vi "Main.vi"() -> ()   [LabVIEW 2024]
doc: "This sample project is built upon the standard state machine template and shows how you could create an application that acquires, analyzes, and presents data. It includes functionality for presenting configuration dialogs, preserving settings between executions, loading and saving data, as well as exporting graph images and text files.\n\nIt is most appropriate for data that is acquired instantly as it does not allow for screen updates mid acquisition nor does it allow for continuous streaming to disk."
uses:
  controls/Vac Graph Config.ctl
  controls/TestCycleParams.ctl
  controls/SurviveCycleParams.ctl
  controls/ControlInput.ctl
  controls/PID Params.ctl
  controls/State.ctl
  <vilib>/Platform/TimedLoop/XDataNode/timing_clust.ctl
  <vilib>/Platform/TimedLoop/XDataNode/nitl_modes.ctl
  <vilib>/Platform/TimedLoop/XDataNode/wakeup.ctl
  <vilib>/platform/TimedLoop/XDataNode/XDataNode.xnode
  <instrlib>/PL Inficon VGC/PL Inficon VGC.lvclass
  <vilib>/Platform/TimedLoop/XDataNode/XDNodeRunTimeDep.lvlib
  <instrlib>/Stanford PTC10/SRS PTC10.lvlib
  <userlib>/_OpenG.lib/time/time.llb/openg_time.lvlib
panel:
  in  "Save Settings on exit":bool=TRUE
  in  "Load Settings":bool
  in  "Save Settings":bool
  out "stopping":bool=TRUE
  in  "Exit":bool
  in  "Main Tabs":enum32{"Setup", "Operating", "ExportData"}(tab)
  in  "Hardware Setup Tabs":T1(tab)=enum."Temperature Control"
  in  "Chamber SP":T2={"mode"=3, "thresholds"={"lower"=0.0001, "upper"=0.0005}, "on"=TRUE} {"thresholds"."upper" format="%#_5e"; "thresholds"."lower" format="%#_5g"; "mode" items=["off", "on", "channel 1", "channel 2", "channel 3"]}
  in  "Backing SP":T2={"mode"=2, "thresholds"={"lower"=1.0, "upper"=5.0}, "on"=TRUE} {"thresholds"."upper" format="%#_5g"; "thresholds"."lower" format="%#_5g"; "mode" items=["off", "on", "channel 1", "channel 2", "channel 3"]}
  out "device information":T3={"type"="VGC503", "model number"="398-483", "serial number"="7433", "firmware version"="1.07", "hardware version"="1.0"}
  out "Cycle Preview":cluster{dbl[], dbl[]}(graph)
  in  "TestCycleParameters":T4={"TAmb"=20.0, "HeaterTestTemp"=-80.0, "HeaterTestDwell"=30, "HeaterTestDuration"=15, "MinOpTemp"=-50.0, "MinOpDwell(min)"=30, "TestHeatingRate (deg/min)"=0.4, "SurviveCycleParameters"={"MinSurviveTemp"=-131.5, "MinSurvive Dwell"=10, "MaxOpTemp"=50.0, "MaxOpDwell"=30, "ControlInput"=2, "ColdStandOff"=4.0, "HotStandoff"=5.0, "SteadyPWM"=20, "MaxCoolingRate (deg/min)"=3.75, "MaxHeatingRate (deg/min)"=2.5}, "CycleType"=0} {"CycleType" items=["Survival", "Operational"]; "SurviveCycleParameters"."SteadyPWM" min=0 max=100 step=1; "SurviveCycleParameters"."ControlInput" items=["3A", "3B", "3C", "3D", "4A", "4B", "4C", "4D"]}
  in  "PTC setup Tabs":enum32{"Macros", "Channels"}(tab)
  in  "PTC Macro Tabs":T7(tab)=enum."ToAmbient"
  out "pwmloop":string="define pwmloop(#t=0 while (1) {waitforsample if(#pwm=0){relays=0}else{if(#t<#pwm) {relays=1}else{relays=3}}#t+=1 if  (#t>99){#t=0} pause 0.2 s})"
  out "Stat1":bool=TRUE
  out "onecycle Macro":string="define onecycle (pwm=100 run pwmloop 5A.PID.Setpoint=-130.0 5A.PID.input=3C while(#3C>-129.0){pause 0.2 s}pwm=10 pause 100 min pwm=0  5A.PID.SetPoint=50.0 while(#3C<49.0){pause 0.2 s} pause 10 min kill pwmloop)"
  out "Stat2":bool=TRUE
  out "control":string="define control (while (#Cycles>0) {onecycle pause 1 s #Cycles-=1})"
  out "Stat3":bool=TRUE
  out "HeatDrive":string="define Failsafe (while(1) {if (#Check <-20){pwm=0 relays=0 outputEnable Off}else{if(#Check>20){pwm=0 relays=0 outputEnable Off}} pause 1 s})"
  out "Stat4":bool=TRUE
  out "ToAmbient":string="define Failsafe (while(1) {if (#Check <-20){pwm=0 relays=0 outputEnable Off}else{if(#Check>20){pwm=0 relays=0 outputEnable Off}} pause 1 s})"
  out "Stat5":bool=TRUE
  in  "TAmbient":dbl=20.0 min=0.0 max=30.0
  in  "AmbientTolerance":dbl=5.0
  out "Startup Code":string
  in  "PTC Channels":enum32{"Heater Output", "Alarm"}(tab)
  out "Control Input":string
  in  "PID Params":T8={"P"=1.14, "I"=0.012, "D"=21.68} {"D" min=0.0; "I" min=0.0; "P" min=0.0}
  in  "Send to PTC":bool
  out "Response":string
  in  "Command":string
  out "PTC10 Info":T9={"Manufacturer"="Stanford Research Systems", "Instrument"=" PTC10 Programmable Temperature Controller", "Serial Number"=" 153826", "Firmware"=" version 4.56"}
  out "Event log":string
  in  "Enable":bool
  in  "Log Interval (s)":dbl=5.0 min=0.1 max=100.0
  in  "LogFile":path=path "C:/Users/Public/Documents/TVC Logs/platten1.xlsx"
  out "Application:Kind":T10(ring)
  out "App Version":string
  out "CycleNumber":i32
  in  "ToTarget":bool
  in  "Target":dbl
  in  "Start":bool
  in  "Cycles to \nPerform":i32=1 min=1 max=1000 step=1
  out "Current \nTarget\nTemperature":dbl=50.0
  in  "Operating Tabs":enum32{"Vacuum", "Temperatures", "Heater Drive"}(tab)
  out "Pressures":waveform(dbl)[](graph)
  out "Backing Good":bool=TRUE
  out "Chamber Good":bool=TRUE
  in  "Vacuum Graph config":T11={"Log/Lin"=TRUE, "Show Backing"=TRUE, "Show Chamber"=TRUE}
  in  "Clear Vacuum Chart":bool
  in  "Clear Charts":bool
  out "Temperature Chart":dynamicdata(graph)
  out "Heater Drive":waveform(dbl)(graph)
  out "Cycles Remaining":i16=1 caption="Cycles\nRemaining"
  out "Relays":T12
  out "Relay wfm":waveform(dbl)
  out "TVC_temperatures_wfm":waveform(dbl)[](array[waveform])
  out "TVC_Temperatures":dbl[](array[numeric])
  out "Status Bar":string="Application exit."
  # "The FileSafe macro looks at the \"Check\" channel every second.\nIf the value is greater than 20, the macro with disable outputs and switch off the cold head."
  # "The heater output channel (5A) provides an analog control voltage\nto the constant current programming input on the CPX400SA \npower supply.\n\nThe Control Input is the RTD input channel that controls the PID loop.\n\nSetup so that 2V output(maximum) corresponds to approx 4A\nof heater current.\n\nSet PID parameters"
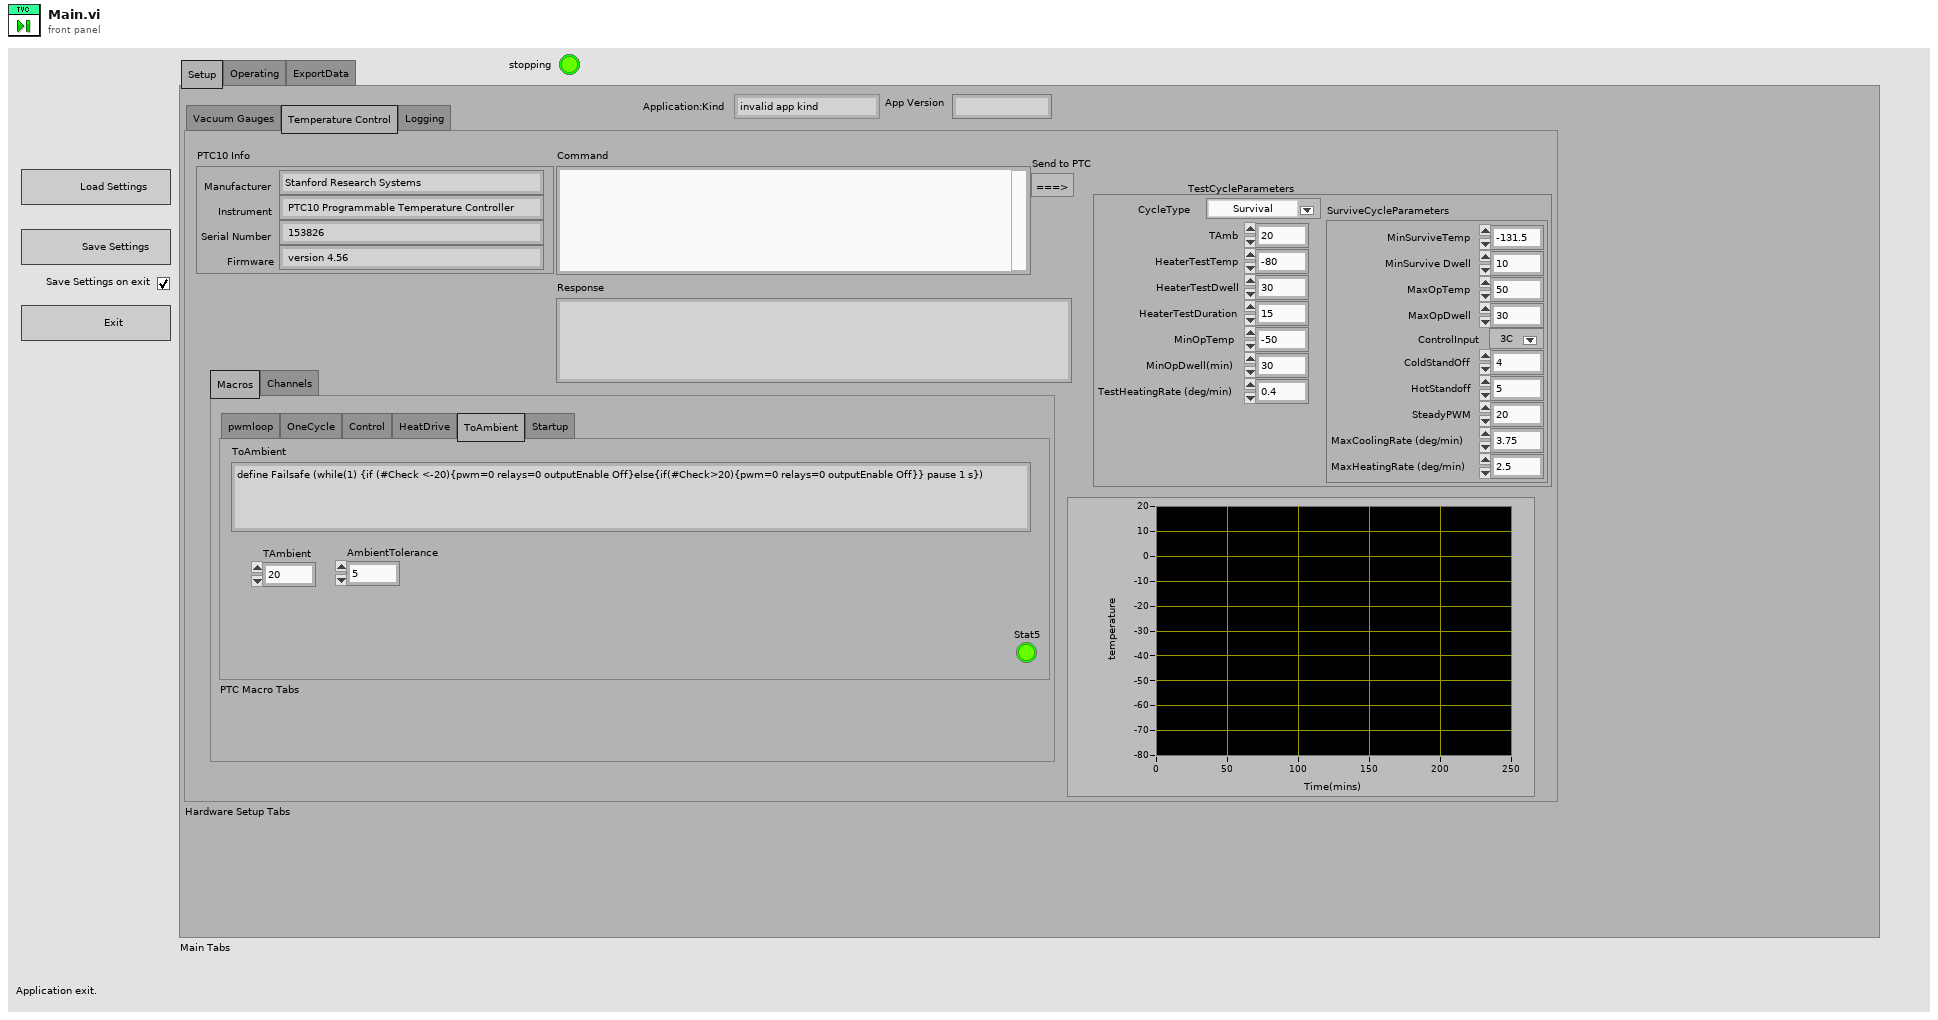
[diagram p1: front panel]
types:
  T1 = enum32{"Vacuum Gauges", "Temperature Control", "Logging"}
  T2 = cluster{"mode":u16, "thresholds":cluster{"lower":dbl, "upper":dbl}, "on":bool}
  T3 = cluster{"type":string, "model number":string, "serial number":string, "firmware version":string, "hardware version":string}
  T4 = typedef "TestCycleParams.ctl" = cluster{"TAmb":dbl, "HeaterTestTemp":dbl, "HeaterTestDwell":i32, "HeaterTestDuration":i32, "MinOpTemp":dbl, "MinOpDwell(min)":i32, "TestHeatingRate (deg/min)":dbl, "SurviveCycleParameters":T5, "CycleType":u16}
  T5 = typedef "SurviveCycleParams.ctl" = cluster{"MinSurviveTemp":dbl, "MinSurvive Dwell":i32, "MaxOpTemp":dbl, "MaxOpDwell":i32, "ControlInput":T6, "ColdStandOff":dbl, "HotStandoff":dbl, "SteadyPWM":i32, "MaxCoolingRate (deg/min)":dbl, "MaxHeatingRate (deg/min)":dbl}
  T6 = typedef "ControlInput.ctl" = u16
  T7 = enum32{"pwmloop", "OneCycle", "Control", "HeatDrive", "ToAmbient", "Startup"}
  T8 = typedef "PID Params.ctl" = cluster{"P":dbl, "I":dbl, "D":dbl}
  T9 = cluster{"Manufacturer":string, "Instrument":string, "Serial Number":string, "Firmware":string}
  T10 = enum32{"invalid app kind", "Development System", "Run Time System", "Student Edition", "Embedded LabVIEW", "Evaluation", "Custom"}
  T11 = typedef "Vac Graph Config.ctl" = cluster{"Log/Lin":bool, "Show Backing":bool, "Show Chamber":bool}
  T12 = cluster{"Sys ON":bool, "Cold Pause":bool, "Alarm":bool}
  T13 = typedef "State.ctl" = enum16{"Initialize", "InitHardware", "WritePTCCode", "CodeToPTC", "Wait for Event", "Update UI", "Save Settings", "Load Settings", "ShutDownHardware", "Exit"}
  T14 = typedef "Data.ctl" = cluster{"UI References":T15, "User Specified":T16}
  T15 = typedef "UI References.ctl" = cluster{"Exit Ref":refnum<vi>, "Save Ref":refnum<vi>, "Export Ref":refnum<vi>, "Acquire Ref":refnum<vi>, "Configure Ref":refnum<vi>, "Graph Ref":refnum<vi>, "Analyze Ref":refnum<vi>, "Status Ref":refnum<vi>, "Snapshot Ref":refnum<vi>, "Start Ref":refnum<vi>}
  T16 = typedef "User Specified Data.ctl" = cluster{"Hardware Configuration":T17, "Vacuum Graph config":T11}
  T17 = typedef "HW Configuration.ctl" = cluster{"VGC50":T18, "PTC10":T19}
  T18 = typedef "VGC50.ctl" = cluster{"serial settings":cluster{"port":refnum<visa-resource-name>, "baud rate":u32}, "device information":cluster{"type":string, "model number":string, "serial number":string, "firmware version":string, "hardware version":string}, "VGC":refnum<class "PL Inficon VGC.lvclass">, "Backing SP":cluster{"mode":u16, "thresholds":cluster{"lower":dbl, "upper":dbl}, "on":bool}, "Chamber SP":cluster{"mode":u16, "thresholds":cluster{"lower":dbl, "upper":dbl}, "on":bool}}
  T19 = typedef "SRS PTC10.ctl" = cluster{"serial settings":cluster{"port":refnum<visa-resource-name>, "baud rate":u32}, "PTC10 Info":cluster{"Manufacturer":string, "Instrument":string, "Serial Number":string, "Firmware":string}, "VISA resource name":refnum<visa-resource-name>, "pwmloop":string, "onecycle":string, "control":string, "HeatDrive":string, "ToAmbient":string, "StartupCode":string, "LogChannels":string[], "Heater O/P Channel":string, " Control Input":string, "TAmbient":dbl, "AmbientTolerance":dbl, "TestCycleParameters":T4, "PID Params":T8}
  T20 = enum8{"Expect success", "Expect error", "Don't check for err"}
  T21 = cluster{"Boolean array[0]":bool, "Boolean array[1]":bool, "Boolean array[2]":bool}
  T22 = typedef "XDNodeRunTimeDep.lvlib/timing_clust.ctl" = cluster{"Expected End [f-1]":u64, "Actual End [f-1]":u64, "Finished Late? [f-1]":bool, "Expected End [i-1]":u64, "Actual End [i-1]":u64, "Finished Late? [i-1]":bool, "Expected Start [i]":u64, "Actual Start [i]":u64, "Expected Start [f]":u64, "Actual Start [f]":u64, "Source Name":string, "Structure Name":string, "Period":i64, "Deadline":i64, "Offset":i64, "Start":i64, "Priority":i32, "Timeout":i32, "Mode":T23, "Wakeup Reason":T24, "Error":errorcluster, "Source Type":string, "Secondary Source Type":string, "Global End Time":u64, "Global Start Time":u64, "Frame Duration":u64, "Iteration Duration":u64, "Assigned CPU":i32, "I/O Scan Engine Mode":u32}
  T23 = typedef "XDNodeRunTimeDep.lvlib/nitl_modes.ctl" = enum32{"No Change", "Process missed periods, maintain original phase", "Discard missed periods, maintain original phase", "Process missed periods, ignore original phase", "Discard missed periods, ignore original phase"}
  T24 = typedef "XDNodeRunTimeDep.lvlib/wakeup.ctl" = enum32{"Normal", "Aborted", "Asynchronous wakeup", "Timing source error", "Timed loop error", "Timeout"}
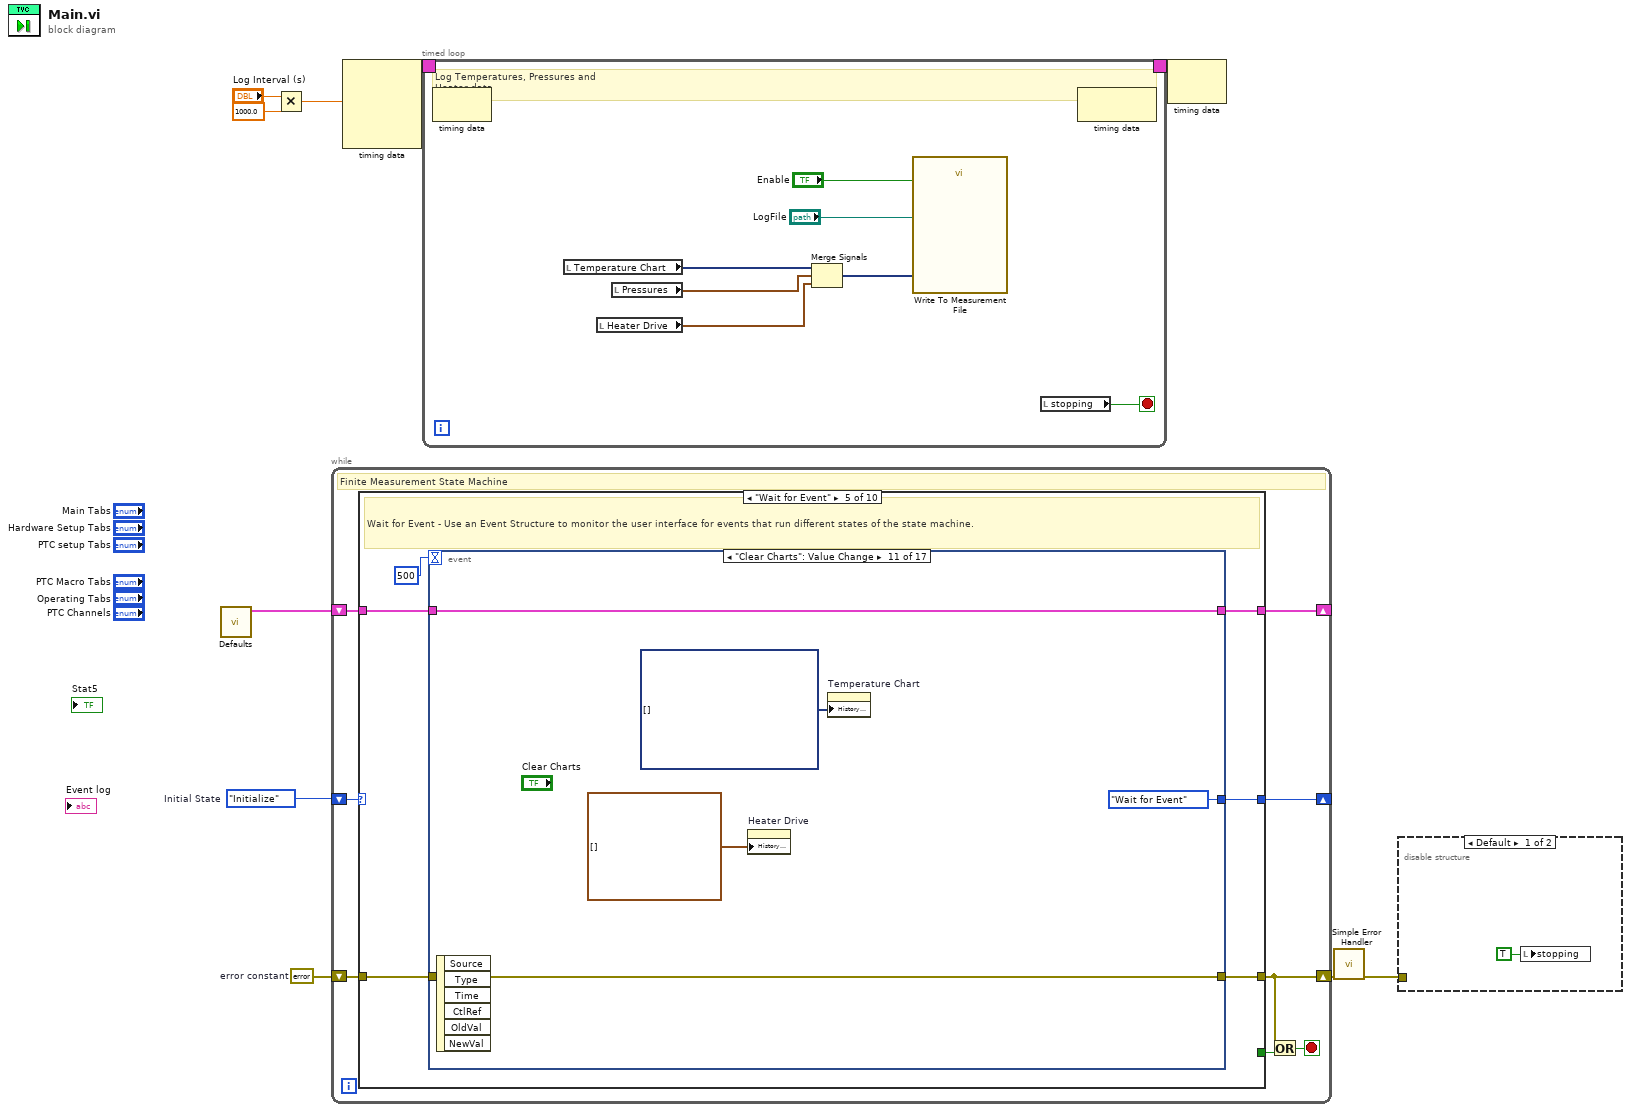
[diagram p0: block diagram]
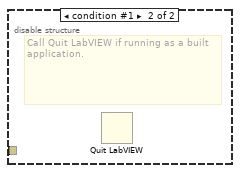
[diagram p2: hidden frame]
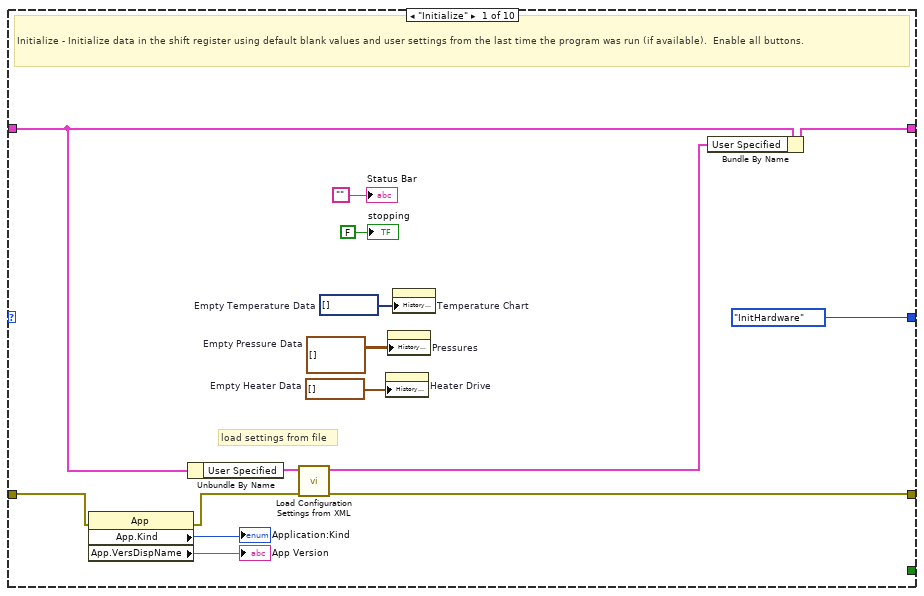
[diagram p3: hidden frame]
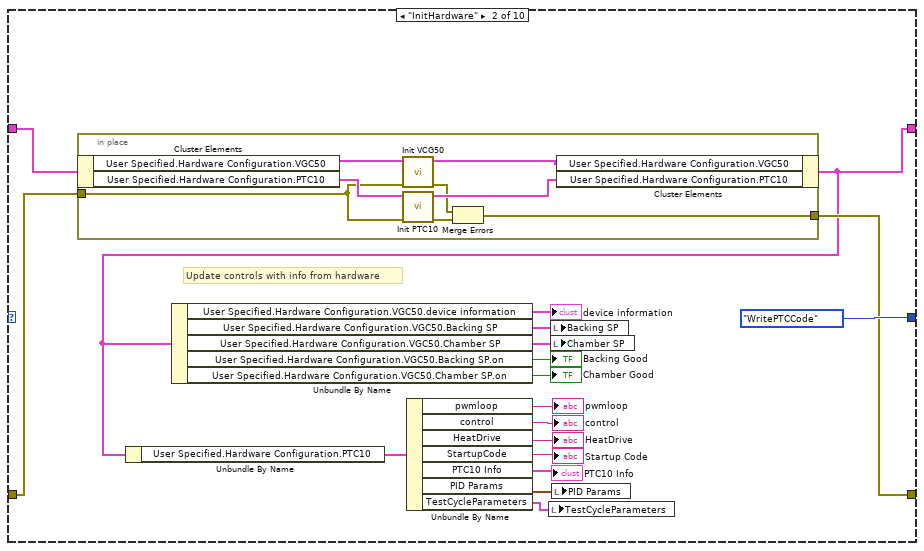
[diagram p4: hidden frame]
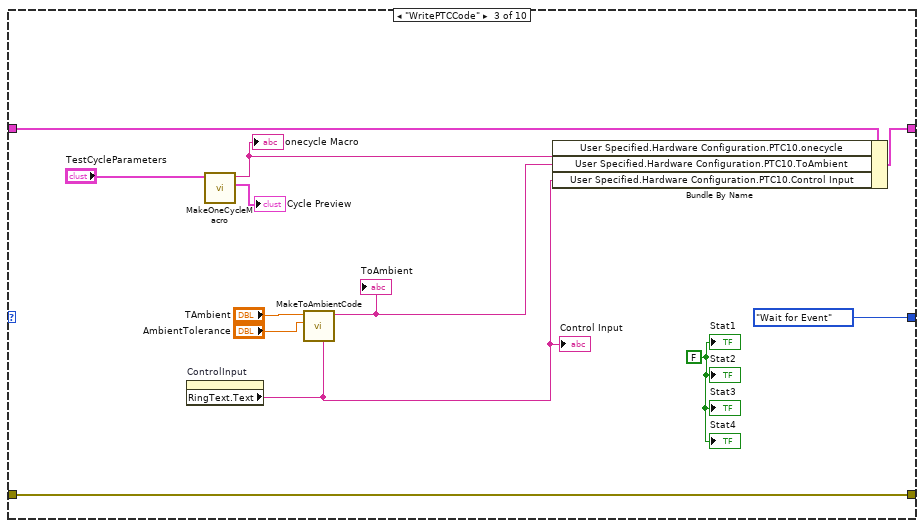
[diagram p5: hidden frame]
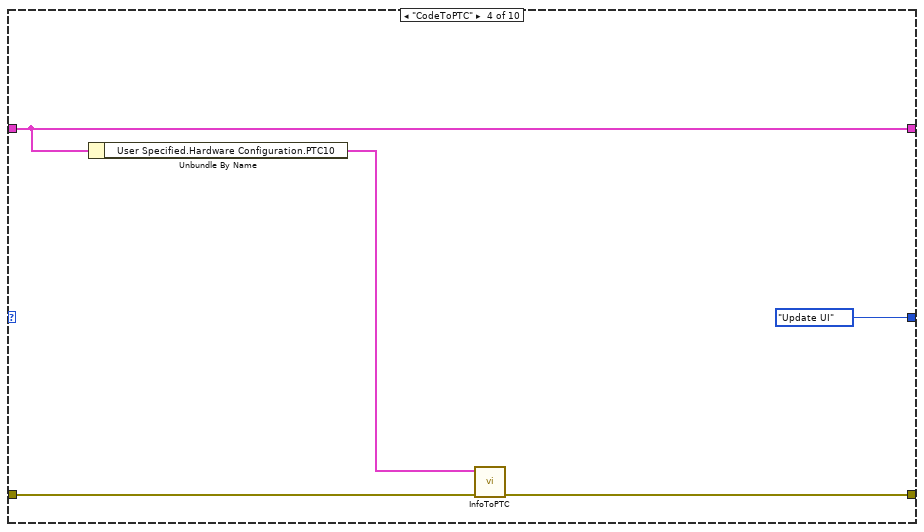
[diagram p6: hidden frame]
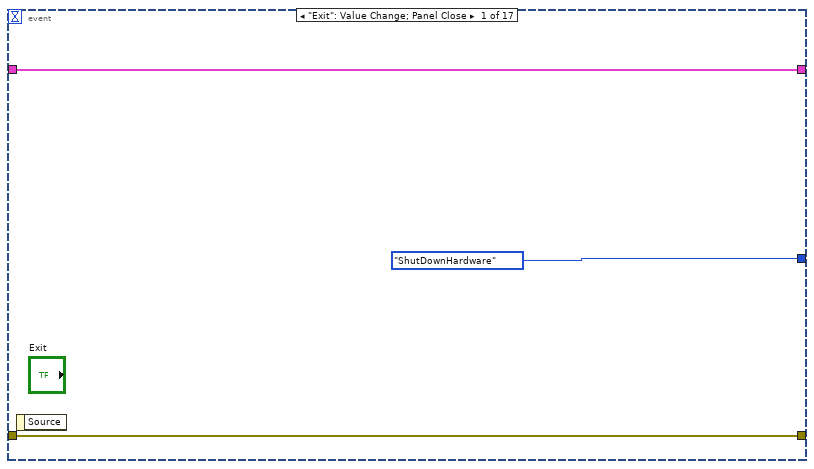
[diagram p7: hidden frame]
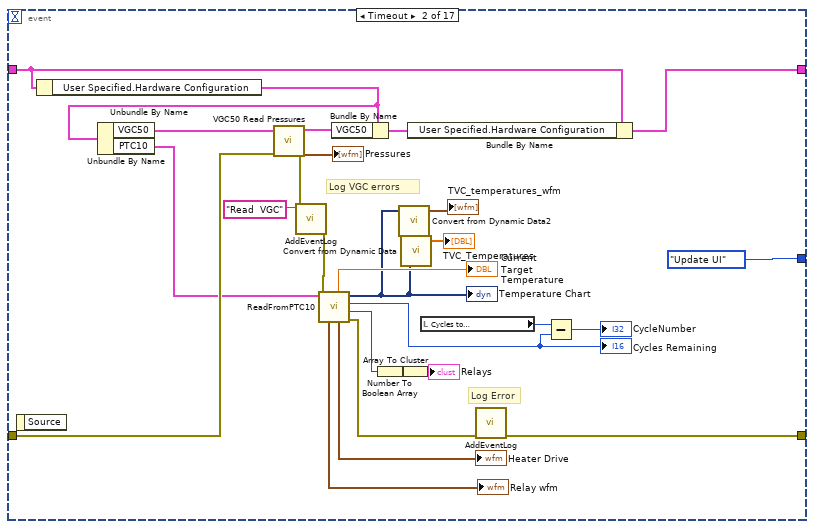
[diagram p8: hidden frame]
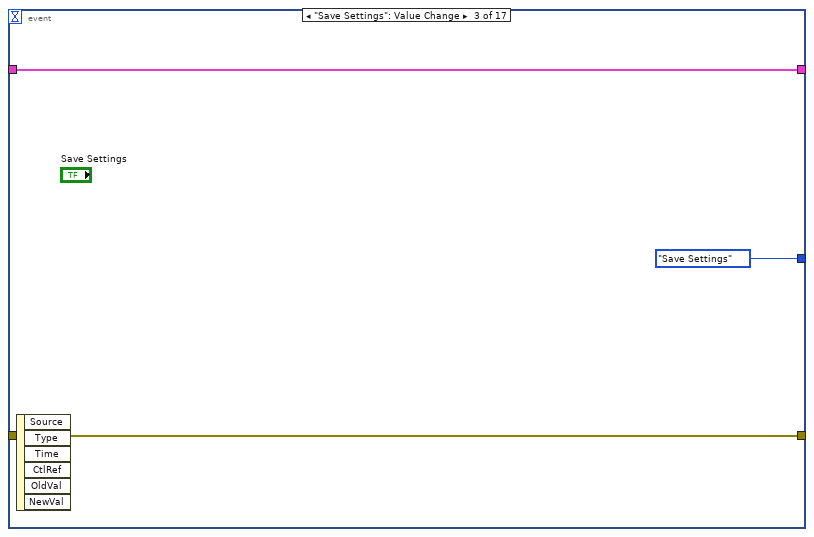
[diagram p9: hidden frame]
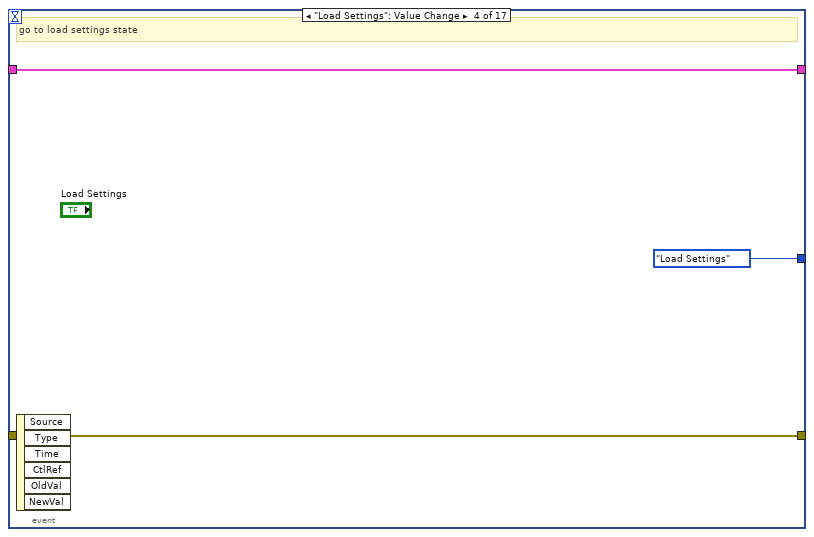
[diagram p10: hidden frame]
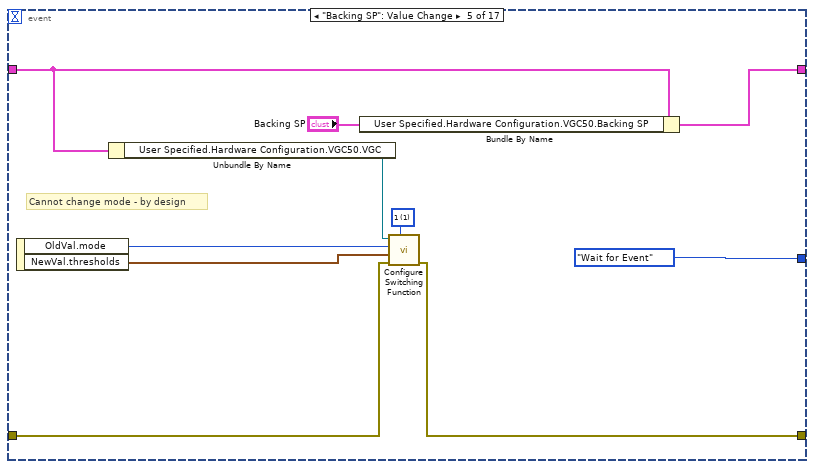
[diagram p11: hidden frame]
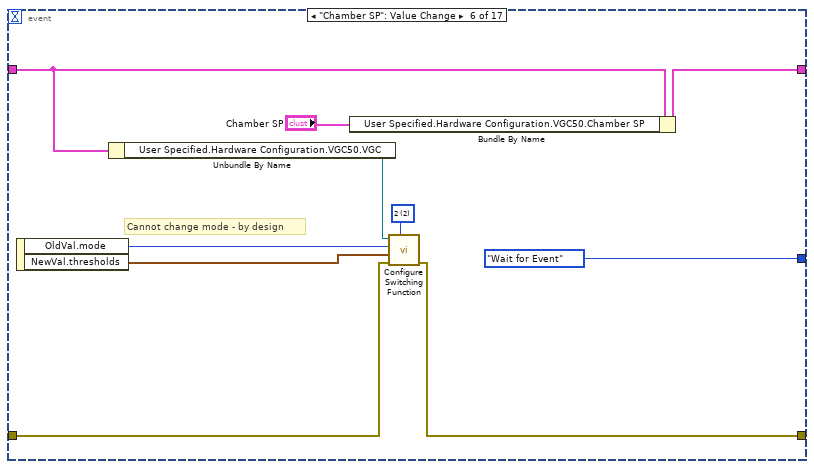
[diagram p12: hidden frame]
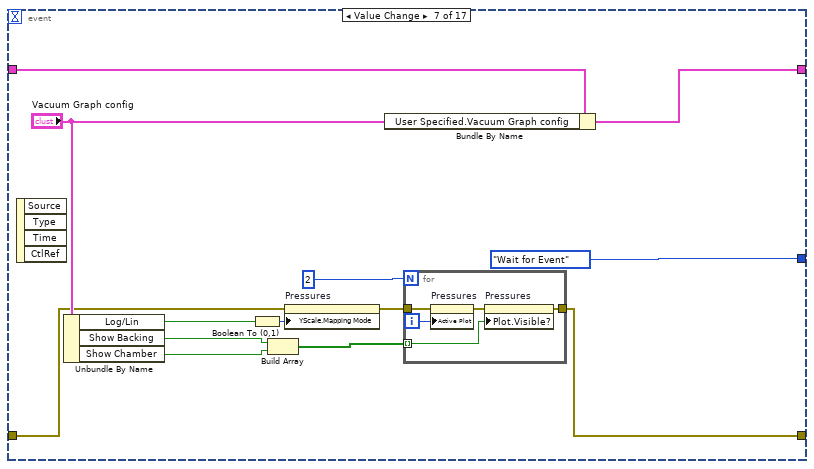
[diagram p13: hidden frame]
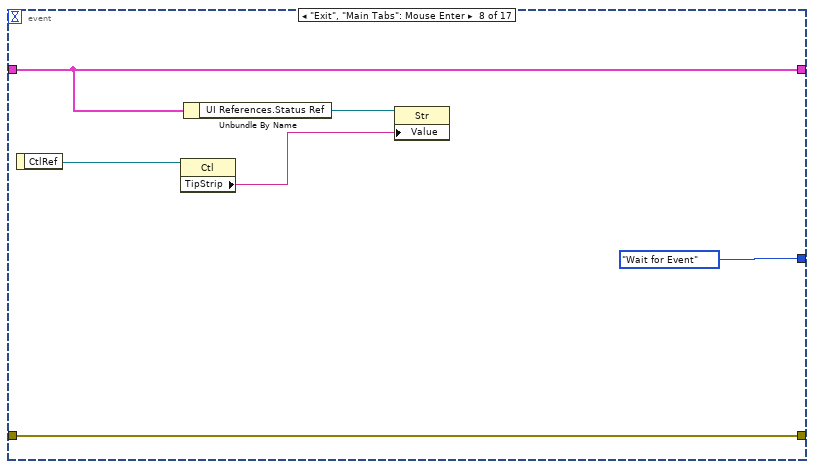
[diagram p14: hidden frame]
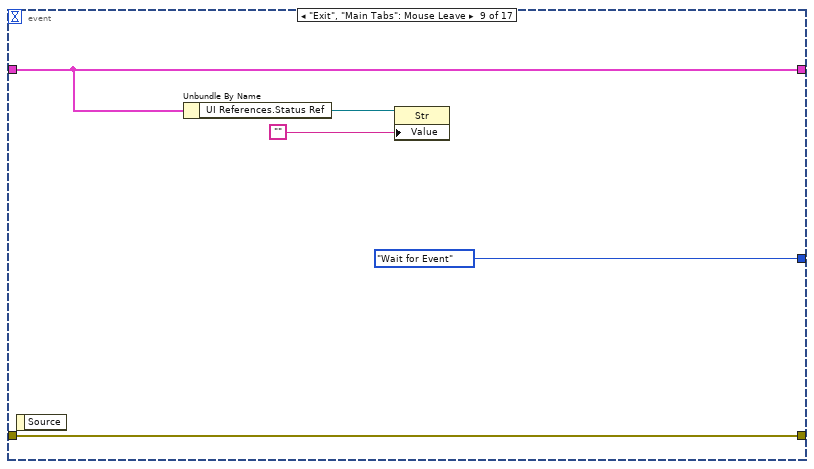
[diagram p15: hidden frame]
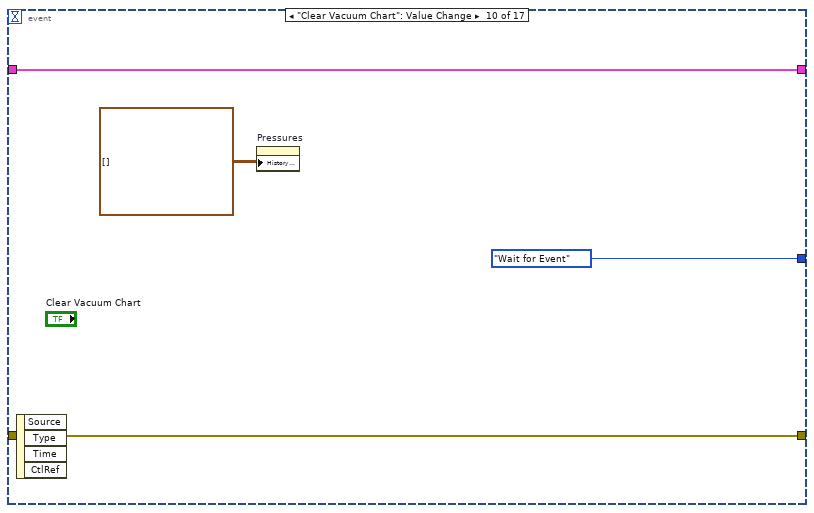
[diagram p16: hidden frame]
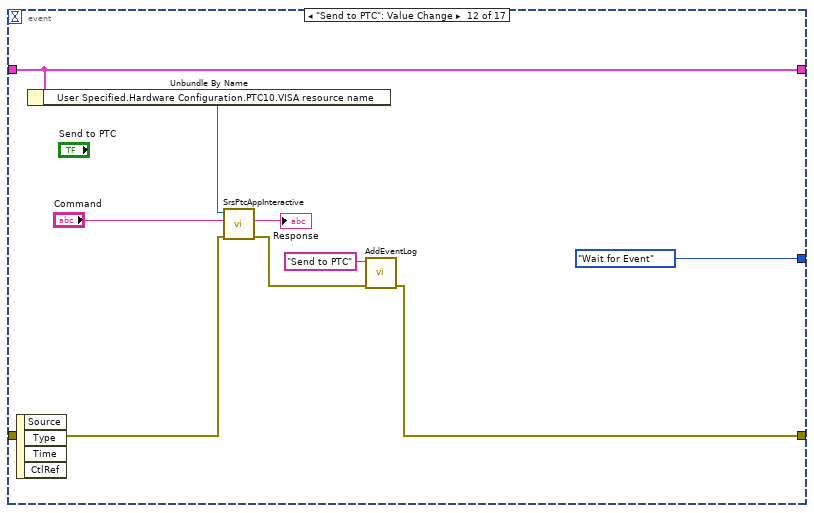
[diagram p17: hidden frame]
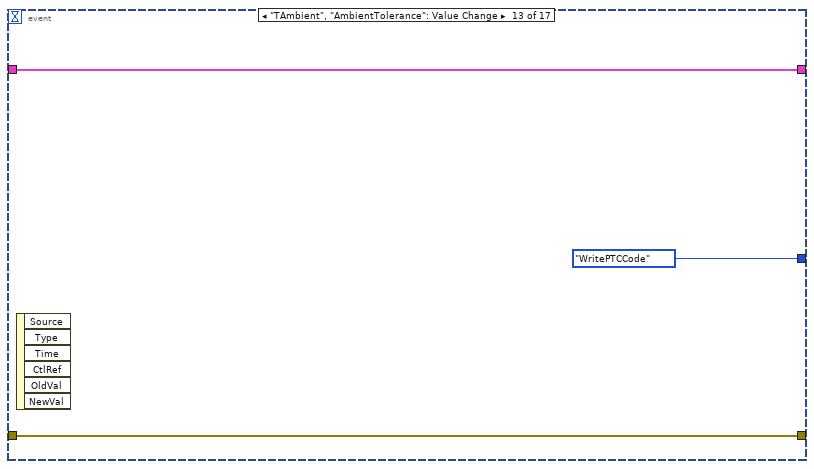
[diagram p18: hidden frame]
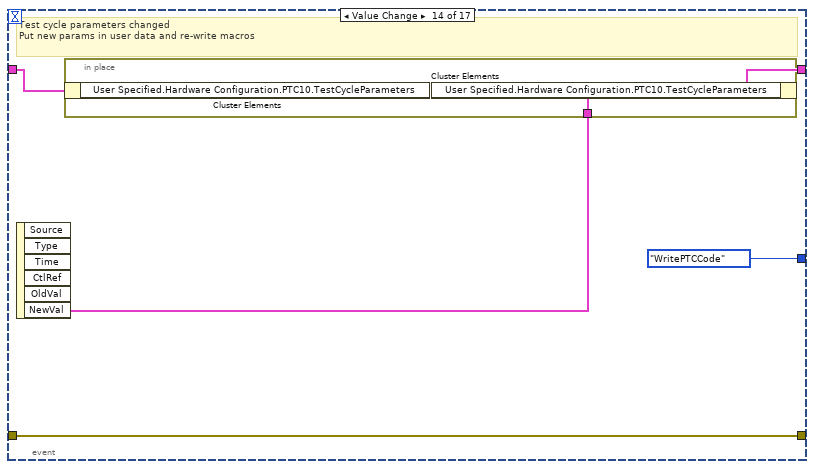
[diagram p19: hidden frame]
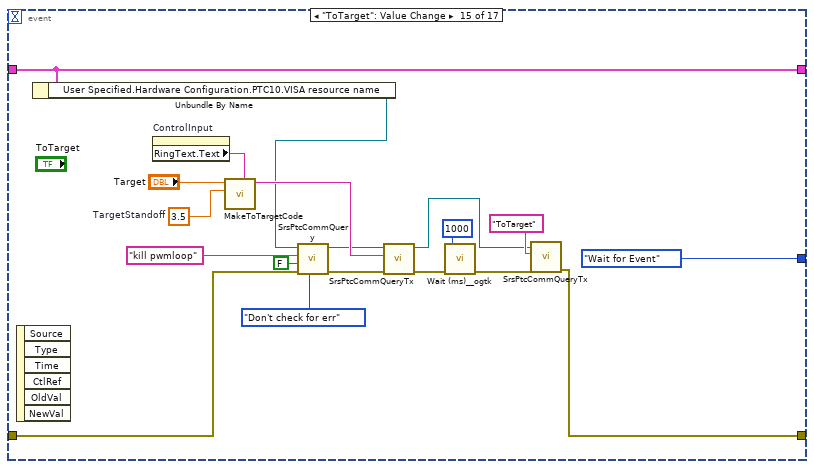
[diagram p20: hidden frame]
diagram:
  w9 = errorcluster {"status"=FALSE, "code"=0, "source"=""}  # error constant
  w10 = State."Initialize"  # Initial State
  n1 = call "Defaults.vi"() -> ("TVC Data"=w6:T14)  [unwired: 11 in]
  n2 = Multiply(x="Log Interval (s)", y=1000.0) -> (x*y=w1:dbl)
  n3 = while {
    shift-right: [w17] -> _
    shift-left: w10 -> [w18]
    shift-right: [w15] -> _
    shift-left: w6 -> [w16]
    shift-right: [w11] -> w8
    shift-left: w9 -> [w14]
    stop <- w12 stop-if-true
    # "Finite Measurement State Machine"
    n4 = case shown="\"Wait for Event\"" w18 {
      tunnel: [State."InitHardware" ("Next State") State."WritePTCCode" ("(Value Not Used)") State."Wait for Event" ("(Value Not Used)") State."Update UI" ("(Value Not Used)") w82 State."Wait for Event" ("(Value Not Used)") State."Exit" ("(Value Not Used)") State."Wait for Event" ("(Value Not Used)") State."Wait for Event" ("(Value Not Used)") w294] -> w17
      tunnel: [_ _ _ _ _ _ _ _ _ w293] -> w13
      tunnel: w16 -> [w32 w36 w62 w75 w81 w247 w261 w267 w280 w292]
      tunnel: [w27 w35 w68 w75 w80 w247 w261 w267 w268 w292] -> w15
      tunnel: w14 -> [w24 w50 w71 w73 w79 w249 w251 w265 w279 w289]
      tunnel: [w31 w49 w71 w72 w78 w249 w250 w264 w278 w288] -> w11
      frame "Initialize" {
        w19 = waveform(dbl)[] []  # Empty Heater Data
        w20 = waveform(dbl)[][] []  # Empty Pressure Data
        w21 = dynamicdata[] []  # Empty Temperature Data
        # "load settings from file"
        # "Initialize - Initialize data in the shift register using default blank values and user settings from the last time the program was run (if available).  Enable all buttons."
        n5 = property class="App"(error in=w24) -> (error out=w25:errorcluster, "App.Kind"=→"Application:Kind":T10, "App.VersDispName"=→"App Version":string)  [unwired: 1 in, 1 out]
        n6 = Unbundle By Name(w32) -> ("User Specified"=w28:T16)
        n7 = call "Load Configuration Settings from XML.vi"("error in (no error)"=w25, "User Specified"=w28) -> ("error out"=w31:errorcluster, "User Specified Out"=w26:T16)  [unwired: 8 in]
        n8 = property on="Heater Drive" class="WFChart (strict)"("History Data"=w19) -> ()  [unwired: 2 in, 2 out]
        n9 = property on="Pressures" class="WFChart (strict)"("History Data"=w20) -> ()  [unwired: 2 in, 2 out]
        n10 = property on="Temperature Chart" class="WFChart (strict)"("History Data"=w21) -> ()  [unwired: 2 in, 2 out]
        n11 = Bundle By Name(cluster=w32, "User Specified"=w26) -> (w27:T14)
        "Status Bar" <- "" ("Status Bar")
        "stopping" <- FALSE ("stopping")
      }
      frame "InitHardware" {
        # "Update controls with info from hardware"
        n12 = in-place {
          in-place-border: w50 -> [w54]
          in-place-border: [w53] -> w49
          n13 = in-place-cluster #1(w36) -> ("User Specified.Hardware Configuration.VGC50"=w59:T18, "User Specified.Hardware Configuration.PTC10"=w57:T19)
          n14 = call "Init VCG50.vi"("error in (no error)"=w54, "VGC50 In"=w59) -> ("error out"=w52:errorcluster, "VGC50 Out"=w58:T18)  [unwired: 8 in]
          n15 = call "Init PTC10.vi"("error in (no error)"=w54, "PTC10"=w57) -> ("error out"=w55:errorcluster, "PTC10 Out"=w56:T19)  [unwired: 8 in]
          n16 = Merge Errors(w52, w55) -> (w53:errorcluster)
          n17 = in-place-cluster #1("User Specified.Hardware Configuration.VGC50"=w58, "User Specified.Hardware Configuration.PTC10"=w56) -> (w35:T14)
        }
        n18 = Unbundle By Name(w35) -> ("User Specified.Hardware Configuration.PTC10"=w39:T19)
        n19 = Unbundle By Name(w35) -> ("User Specified.Hardware Configuration.VGC50.device information"=→"device information":T3, "User Specified.Hardware Configuration.VGC50.Backing SP"=w47:T2, "User Specified.Hardware Configuration.VGC50.Chamber SP"=w46:T2, "User Specified.Hardware Configuration.VGC50.Backing SP.on"=→"Backing Good":bool, "User Specified.Hardware Configuration.VGC50.Chamber SP.on"=→"Chamber Good":bool)
        n20 = Unbundle By Name(w39) -> ("pwmloop"=→"pwmloop":string, "control"=→"control":string, "HeatDrive"=→"HeatDrive":string, "StartupCode"=→"Startup Code":string, "PTC10 Info"=→"PTC10 Info":T9, "PID Params"=w37:T8, "TestCycleParameters"=w34:T4)
        n21 = local write "TestCycleParameters"(w34) -> ()
        n22 = local write "Backing SP"(w47) -> ()
        n23 = local write "Chamber SP"(w46) -> ()
        n24 = local write "PID Params"(w37) -> ()
      }
      frame "WritePTCCode" {
        w69 = FALSE ("Stat1")
        n25 = property on="ControlInput" class="Ring (strict)"() -> ("RingText.Text"=w61:string)  [unwired: 2 in, 2 out]
        "Control Input" <- w61
        n26 = call "MakeOneCycleMacro.vi"("TestCycleParameters"="TestCycleParameters") -> ("Profile Graph"=→"Cycle Preview":cluster{dbl[], dbl[]}, "Macro Code"=w60:string)  [unwired: 9 in]
        "onecycle Macro" <- w60
        n27 = call "MakeToAmbientCode.vi"("ControlInput"=w61, "AmbientTolerance"="AmbientTolerance", "TAmbient"="TAmbient") -> ("ToAmbient"=w65:string)  [unwired: 8 in]
        "ToAmbient" <- w65
        n28 = Bundle By Name(cluster=w62, "User Specified.Hardware Configuration.PTC10.onecycle"=w60, "User Specified.Hardware Configuration.PTC10.ToAmbient"=w65, "User Specified.Hardware Configuration.PTC10.Control Input"=w61) -> (w68:T14)
        "Stat2" <- w69
        "Stat1" <- w69
        "Stat3" <- w69
        "Stat4" <- w69
      }
      frame "CodeToPTC" {
        n29 = Unbundle By Name(w75) -> ("User Specified.Hardware Configuration.PTC10"=w74:T19)
        n30 = call "InfoToPTC.vi"("error in (no error)"=w73, "PTC10"=w74) -> ("error out"=w72:errorcluster)  [unwired: 9 in]
      }
      frame "Wait for Event" {
        # "Wait for Event - Use an Event Structure to monitor the user interface for events that run different states of the state machine."
        n31 = event shown="[10] \"Clear Charts\": Value Change" {
          selector: _ -> [_ _ _ _ _ _ _ _ _ _ _ _ _ _ _ _ _]
          dyn-events: _ -> [_ _ _ _ _ _ _ _ _ _ _ _ _ _ _ _ _]
          timeout: 500 -> [_ _ _ _ _ _ _ _ _ _ _ _ _ _ _ _ _]
          tunnel: [State."ShutDownHardware" ("Next State") State."Update UI" ("Next State") State."Save Settings" ("Next State") State."Load Settings" ("Next State") State."Wait for Event" ("Next State") State."Wait for Event" ("Next State") State."Wait for Event" ("Next State") State."Wait for Event" ("Next State") State."Wait for Event" ("Next State") State."Wait for Event" ("Next State") State."Wait for Event" ("Next State") State."Wait for Event" ("Next State") State."WritePTCCode" ("Next State") State."WritePTCCode" ("Next State") State."Wait for Event" ("Next State") State."Wait for Event" ("Next State") State."Wait for Event" ("Next State")] -> w82
          tunnel: w81 -> [w84 w110 w115 w118 w128 w138 w149 w160 w166 w169 w176 w184 w188 w192 w213 w216 w245]
          tunnel: [w84 w109 w115 w118 w127 w137 w148 w160 w166 w169 w176 w184 w188 w190 w213 w216 w246] -> w80
          tunnel: w79 -> [w83 w111 w114 w117 w125 w136 w140 w162 w167 w171 w175 w180 w187 w193 w202 w218 w238]
          tunnel: [w83 w98 w114 w117 w121 w131 w139 w162 w167 w171 w175 w177 w187 w193 w208 w214 w244] -> w78
          event "Exit": Value Change; Panel Close {
            n32 = event-data() -> ()  [unwired: 1 in, 1 out]
          }
          event Timeout {
            # "Log VGC errors"
            # "Log Error"
            n33 = event-data() -> ()  [unwired: 1 in, 1 out]
            n34 = Unbundle By Name(w110) -> ("User Specified.Hardware Configuration"=w106:T17)
            n35 = Unbundle By Name(w106) -> ("VGC50"=w105:T18, "PTC10"=w104:T19)
            n36 = call "VGC50 Read Pressures.vi"("error in (no error)"=w111, "VGC50 In"=w105) -> ("error out"=w103:errorcluster, "VGC50 Out"=w108:T18, "Waveform Chart"=→"Pressures":waveform(dbl)[])  [unwired: 5 in, 2 out]
            n37 = call "AddEventLog.vi"("error in (no error)"=w103, "Event"="Read  VGC") -> ("error out"=w99:errorcluster)  [unwired: 9 in]
            n38 = call "ReadFromPTC10.vi"("error in (no error)"=w99, "PTC10"=w104) -> ("error out"=w102:errorcluster, "relays"=w100:i8, "Cycles"=w90:i16, "Temperature Chart"=w88:dynamicdata, "HeaterDrive"=→"Heater Drive":waveform(dbl), "Target Temperature"=→"Current \nTarget\nTemperature":dbl, "Relay wfm"=→"Relay wfm":waveform(dbl))  [unwired: 3 in]
            "Temperature Chart" <- w88
            "Cycles Remaining" <- w90
            n39 = Bundle By Name(cluster=w106, "VGC50"=w108) -> (w107:T17)
            n40 = Number To Boolean Array(number=w100) -> (Boolean array=w101:bool[])
            n41 = call "Convert from Dynamic Data2"("Dynamic Data Type"=w88) -> ("Array of Waveform"=→"TVC_temperatures_wfm":waveform(dbl)[])  [unwired: 3 in]
            n42 = Array To Cluster(array=w101) -> (cluster=→"Relays":T21)
            n43 = call "Convert from Dynamic Data"("Dynamic Data Type"=w88) -> ("Array"=→"TVC_Temperatures":dbl[])  [unwired: 3 in]
            n44 = Bundle By Name(cluster=w110, "User Specified.Hardware Configuration"=w107) -> (w109:T14)
            n45 = local read "Cycles to \nPerform"() -> (w91:i32)
            n46 = call "AddEventLog.vi"("error in (no error)"=w102) -> ("error out"=w98:errorcluster)  [unwired: 10 in]
            n47 = Subtract(x=w91, y=w90) -> (x-y=→"CycleNumber":i32)
          }
          event "Save Settings": Value Change {
            n48 = event-data() -> ()  [unwired: 1 in, 6 out]
          }
          event "Load Settings": Value Change {
            # "go to load settings state"
            n49 = event-data() -> ()  [unwired: 1 in, 6 out]
          }
          event "Backing SP": Value Change {
            w122 = u16 1 items=["1"=1, "2"=2, "3"=3, "4"=4, "5"=5, "6"=6] ("function")
            # "Cannot change mode - by design"
            n50 = event-data() -> ("OldVal.mode"=w119:u16, "NewVal.thresholds"=w124:cluster{"lower":dbl, "upper":dbl})  [unwired: 1 in]
            n51 = Unbundle By Name(w128) -> ("User Specified.Hardware Configuration.VGC50.VGC"=w123:refnum<class "PL Inficon VGC.lvclass">)
            n52 = Bundle By Name(cluster=w128, "User Specified.Hardware Configuration.VGC50.Backing SP"="Backing SP") -> (w127:T14)
            n53 = call <instrlib>:"Configure Switching Function.vi"("function"=w122, "error in (no error)"=w125, "thresholds"=w124, "mode"=w119, "VGC in"=w123) -> ("error out"=w121:errorcluster)  [unwired: 3 in, 3 out]
          }
          event "Chamber SP": Value Change {
            w132 = u16 2 items=["1"=1, "2"=2, "3"=3, "4"=4, "5"=5, "6"=6] ("function")
            # "Cannot change mode - by design"
            n54 = event-data() -> ("OldVal.mode"=w134:u16, "NewVal.thresholds"=w135:cluster{"lower":dbl, "upper":dbl})  [unwired: 1 in]
            n55 = Unbundle By Name(w138) -> ("User Specified.Hardware Configuration.VGC50.VGC"=w133:refnum<class "PL Inficon VGC.lvclass">)
            n56 = Bundle By Name(cluster=w138, "User Specified.Hardware Configuration.VGC50.Chamber SP"="Chamber SP") -> (w137:T14)
            n57 = call <instrlib>:"Configure Switching Function.vi"("function"=w132, "error in (no error)"=w136, "thresholds"=w135, "mode"=w134, "VGC in"=w133) -> ("error out"=w131:errorcluster)  [unwired: 3 in, 3 out]
          }
          event Value Change {
            n58 = event-data() -> ()  [unwired: 1 in, 4 out]
            n59 = Unbundle By Name("Vacuum Graph config") -> ("Log/Lin"=w146:bool, "Show Backing"=w144:bool, "Show Chamber"=w143:bool)
            n60 = Boolean To (0,1)(Boolean=w146) -> (0, 1=w151:i16)
            n61 = Build Array(w144, w143) -> (w142:bool[])
            n62 = property on="Pressures" class="WFChart (strict)"(error in=w140, "YScale.Mapping Mode"=w151) -> (error out=w141:errorcluster)  [unwired: 1 in, 1 out]
            n63 = Bundle By Name(cluster=w149, "User Specified.Vacuum Graph config"="Vacuum Graph config") -> (w148:T14)
            n64 = for {
              N: 2 -> [_]
              tunnel: w142 -> [w154] mode=indexing
              tunnel: w141 -> [w153]
              tunnel: [w152] -> w139
              i -> [w155]
              n65 = property on="Pressures" class="WFChart (strict)"(error in=w153, "Active Plot"=w155) -> (error out=w156:errorcluster)  [unwired: 1 in, 1 out]
              n66 = property on="Pressures" class="WFChart (strict)"(error in=w156, "Plot.Visible?"=w154) -> (error out=w152:errorcluster)  [unwired: 1 in, 1 out]
            }
          }
          event "Exit", "Main Tabs": Mouse Enter {
            n67 = event-data() -> ("CtlRef"=w161:refnum<vi>)  [unwired: 1 in]
            n68 = property class="Ctl"(reference=w161) -> ("TipStrip"=w158:string)  [unwired: 1 in, 2 out]
            n69 = Unbundle By Name(w160) -> ("UI References.Status Ref"=w159:refnum<vi>)
            n70 = property class="Str"(reference=w159, "Value"=w158) -> ()  [unwired: 1 in, 2 out]
          }
          event "Exit", "Main Tabs": Mouse Leave {
            n71 = event-data() -> ()  [unwired: 1 in, 1 out]
            n72 = Unbundle By Name(w166) -> ("UI References.Status Ref"=w165:refnum<vi>)
            n73 = property class="Str"(reference=w165, "Value"="") -> ()  [unwired: 1 in, 2 out]
          }
          event "Clear Vacuum Chart": Value Change {
            n74 = event-data() -> ()  [unwired: 1 in, 4 out]
            n75 = property on="Pressures" class="WFChart (strict)"("History Data"=waveform(dbl)[][] []) -> ()  [unwired: 2 in, 2 out]
          }
          event "Clear Charts": Value Change {
            n76 = event-data() -> ()  [unwired: 1 in, 6 out]
            n77 = property on="Heater Drive" class="WFChart (strict)"("History Data"=waveform(dbl)[] []) -> ()  [unwired: 2 in, 2 out]
            n78 = property on="Temperature Chart" class="WFChart (strict)"("History Data"=dynamicdata[] []) -> ()  [unwired: 2 in, 2 out]
          }
          event "Send to PTC": Value Change {
            n79 = event-data() -> ()  [unwired: 1 in, 4 out]
            n80 = Unbundle By Name(w184) -> ("User Specified.Hardware Configuration.PTC10.VISA resource name"=w183:refnum<visa-resource-name>)
            n81 = call <instrlib>:"SrsPtcAppInteractive.vi"("error in"=w180, "Command"="Command", "SRS PTC10 VISA in"=w183) -> ("error out"=w179:errorcluster, "Readback"=→"Response":string)  [unwired: 5 in, 2 out]
            n82 = call "AddEventLog.vi"("error in (no error)"=w179, "Event"="Send to PTC") -> ("error out"=w177:errorcluster)  [unwired: 9 in]
          }
          event "TAmbient", "AmbientTolerance": Value Change {
            n83 = event-data() -> ()  [unwired: 1 in, 6 out]
          }
          event Value Change {
            # "Test cycle parameters changed\nPut new params in user data and re-write macros"
            n84 = event-data() -> ("NewVal"=w191:T4)  [unwired: 1 in, 5 out]
            n85 = in-place {
              in-place-border: w191 -> [w194]
              n86 = in-place-cluster #2(w192) -> ()  [unwired: 1 out]
              n87 = in-place-cluster #2("User Specified.Hardware Configuration.PTC10.TestCycleParameters"=w194) -> (w190:T14)
            }
          }
          event "ToTarget": Value Change {
            w210 = 3.5  # TargetStandoff
            n88 = event-data() -> ()  [unwired: 1 in, 6 out]
            n89 = Unbundle By Name(w213) -> ("User Specified.Hardware Configuration.PTC10.VISA resource name"=w199:refnum<visa-resource-name>)
            n90 = property on="ControlInput" class="Ring (strict)"() -> ("RingText.Text"=w196:string)  [unwired: 2 in, 2 out]
            n91 = call "MakeToTargetCode.vi"("ControlInput"=w196, "TargetStandoff"=w210, "TTarget"="Target") -> ("ToAmbient"=w212:string)  [unwired: 8 in]
            n92 = call <instrlib>:"SrsPtcCommQuery.vi"("Expect error?"=T20."Don't check for err", "error in"=w202, "Timeout is error"=FALSE, "Command"="kill pwmloop", "SRS PTC10 VISA in"=w199) -> ("error out"=w201:errorcluster, "SRS PTC10 VISA out"=w200:refnum<visa-resource-name>)  [unwired: 1 in, 4 out]
            n93 = call <instrlib>:"SrsPtcCommQueryTx.vi"("error in"=w201, "Query"=w212, "SRS PTC10 VISA in"=w200) -> ("error out"=w207:errorcluster, "SRS PTC10 VISA out"=w203:refnum<visa-resource-name>)  [unwired: 6 in, 1 out]
            n94 = call <userlib>:"Wait (ms)__ogtk.vi"("error in (no error)"=w207, "milliseconds to wait"=u32 1000) -> ("error out"=w206:errorcluster)  [unwired: 8 in, 1 out]
            n95 = call <instrlib>:"SrsPtcCommQueryTx.vi"("error in"=w206, "Query"="ToTarget", "SRS PTC10 VISA in"=w203) -> ("error out"=w208:errorcluster)  [unwired: 6 in, 2 out]
          }
          event "Start": Value Change {
            n96 = event-data() -> ()  [unwired: 1 in, 4 out]
            n97 = Unbundle By Name(w216) -> ("User Specified.Hardware Configuration.PTC10"=w215:T19)
            n98 = case shown="True" "Start" {
              tunnel: w218 -> [w220 w237]
              tunnel: w215 -> [_ w230]
              tunnel: [w220 w226] -> w214
              frame False {
              }
              frame True {
                # "1. Stop macros currently running on PTC\n2. Erase existing macros\n3. Upload macros\n4. Set Cycles channel on PTC to desired count\n5. Start Failsafe macro\n6. Enable outputs on PTC\n7. Start Control macro"
                n99 = Unbundle By Name(w230) -> ("VISA resource name"=w229:refnum<visa-resource-name>)
                n100 = call "PTCStopMacros.vi"("error in (no error)"=w237, "PTC10"=w230) -> ("error out"=w236:errorcluster, "PTC10 2"=w235:T19)  [unwired: 8 in]
                n101 = call "PTCDelMacros.vi"("error in (no error)"=w236, "PTC10"=w235) -> ("error out"=w225:errorcluster, "PTC10 2"=w221:T19)  [unwired: 8 in]
                n102 = call "Delay"("error in (no error)"=w225) -> ("error out"=w224:errorcluster)  [unwired: 10 in]
                n103 = call "InfoToPTC.vi"("error in (no error)"=w224, "PTC10"=w221) -> ("error out"=w234:errorcluster)  [unwired: 9 in]
                n104 = call "CyclesToPTC.vi"("Cycles"="Cycles to \nPerform", "error in (no error)"=w234, "PTC10"=w221) -> ("error out"=w232:errorcluster, "PTC10 2"=w231:T19)  [unwired: 7 in]
                n105 = call "RunFailsafe.vi"("error in (no error)"=w232, "PTC10"=w231) -> ("error out"=w223:errorcluster, "PTC10 2"=w222:T19)  [unwired: 8 in]
                n106 = call <instrlib>:"SrsPtcActionOutputEnable.vi"("error in"=w223, "Output Enable"=TRUE, "SRS PTC10 VISA in"=w229) -> ("error out"=w227:errorcluster)  [unwired: 7 in, 1 out]
                n107 = call "RunControl.vi"("error in (no error)"=w227, "PTC10"=w222) -> ("error out"=w226:errorcluster)  [unwired: 8 in, 1 out]
              }
            }
          }
          event Value Change {
            n108 = Unbundle By Name(w245) -> ("User Specified.Hardware Configuration.PTC10.VISA resource name"=w242:refnum<visa-resource-name>)
            n109 = event-data() -> ()  [unwired: 1 in, 6 out]
            n110 = property on="ControlInput" class="Ring (strict)"(error in=w238) -> (error out=w239:errorcluster, "RingText.Text"=w240:string)  [unwired: 1 in, 1 out]
            n111 = Bundle By Name(cluster=w245, "User Specified.Hardware Configuration.PTC10.PID Params"="PID Params") -> (w246:T14)
            n112 = call "Setup PID.vi"("Control Input"=w240, "PID Params"="PID Params", "error in (no error)"=w239, "VISA Refnum in"=w242) -> ("error out"=w244:errorcluster)  [unwired: 6 in, 1 out]
          }
        }
      }
      frame "Update UI" {
        # "Update UI - Update varoious UI element.s depending on state of the system\n\nAt present this is empty, but left in case needed"
      }
      frame "ShutDownHardware" {
        n113 = Unbundle By Name(w261) -> ("User Specified.Hardware Configuration"=w260:T17)
        n114 = Unbundle By Name(w260) -> ("PTC10.VISA resource name"=w252:refnum<visa-resource-name>, "VGC50.VGC"=w259:refnum<class "PL Inficon VGC.lvclass">)  [unwired: 1 out]
        n115 = call <instrlib>:"Close.vi"("error in (no error)"=w251, "VGC in"=w259) -> ("error out"=w256:errorcluster)  [unwired: 9 in]
        n116 = call <vilib>:"Simple Error Handler.vi"("error in (no error)"=w256) -> ("code out"=w257:i32, "error out"=w255:errorcluster)  [unwired: 4 in, 3 out]
        n117 = call <vilib>:"Clear Errors.vi"("error in (no error)"=w255, "specific error code to clear (0: all)"=w257) -> ("error out"=w258:errorcluster)  [unwired: 4 in, 1 out]
        n118 = VISA Close(VISA resource name=w252, error in (no error)=w258) -> (error out=w254:errorcluster)
        n119 = call <vilib>:"Simple Error Handler.vi"("error in (no error)"=w254) -> ("error out"=w253:errorcluster)  [unwired: 4 in, 4 out]
        n120 = call <vilib>:"Clear Errors.vi"("error in (no error)"=w253) -> ("error out"=w250:errorcluster)  [unwired: 5 in, 1 out]
      }
      frame "Save Settings" {
        n121 = Unbundle By Name(w267) -> ("User Specified"=w266:T16)
        n122 = call "Save Configuration Settings to XML.vi"("error in (no error)"=w265, "User Configuration"=w266) -> ("error out"=w264:errorcluster)  [unwired: 9 in]
      }
      frame "Load Settings" {
        n123 = in-place {
          in-place-border: w279 -> [w283]
          in-place-border: [w281] -> w278
          n124 = in-place-cluster #3(w280) -> ("User Specified"=w284:T16)
          n125 = call "Load Configuration Settings from XML.vi"("error in (no error)"=w283, "User Specified"=w284) -> ("error out"=w281:errorcluster, "User Specified Out"=w282:T16)  [unwired: 8 in]
          n126 = in-place-cluster #3("User Specified"=w282) -> (w268:T14)
        }
        n127 = Unbundle By Name(w268) -> ("User Specified.Hardware Configuration.PTC10"=w271:T19)
        n128 = Unbundle By Name(w271) -> ("pwmloop"=w272:string, "control"=w273:string, "HeatDrive"=w274:string, "StartupCode"=w275:string, "PTC10 Info"=w276:T9, "PID Params"=w270:T8, "TestCycleParameters"=w269:T4)
        n129 = local write "pwmloop"(w272) -> ()
        n130 = local write "control"(w273) -> ()
        n131 = local write "HeatDrive"(w274) -> ()
        n132 = local write "Startup Code"(w275) -> ()
        n133 = local write "PTC10 Info"(w276) -> ()
        n134 = local write "PID Params"(w270) -> ()
        n135 = local write "TestCycleParameters"(w269) -> ()
      }
      frame "Exit" {
        w293 = TRUE  # Stop Loop?
        w294 = State."Exit"  # (Value Not Used)
        # "Exit - Saves the user's settings to an XML file and stops execution."
        n136 = Unbundle By Name(w292) -> ("UI References.Status Ref"=w290:refnum<vi>, "User Specified"=w287:T16)
        n137 = local write "stopping"(TRUE ("stopping")) -> ()
        n138 = case shown="False" "Save Settings on exit" {
          tunnel: w289 -> [w295 w298]
          tunnel: [w295 w297] -> w288
          tunnel: w287 -> [_ w296]
          frame False {
          }
          frame True {
            n139 = call "Save Configuration Settings to XML.vi"("error in (no error)"=w298, "User Configuration"=w296) -> ("error out"=w297:errorcluster)  [unwired: 9 in]
          }
        }
        n140 = property class="Str"(reference=w290, "Value"="Application exit." ("Stopped")) -> ()  [unwired: 1 in, 2 out]
      }
    }
    n141 = Or(x=w11, y=w13) -> (x .or. y?=w12:bool)
  }
  n142 = node-c288(w1) -> (w5:T22)  [unwired: 3 in]
  n143 = timed-loop {
    timing: w5 -> [_]
    timing-out: [_] -> w4
    stop <- w304 stop-if-true
    # "Log Temperatures, Pressures and \nHeater data"
    n144 = node-c288() -> ()  [unwired: 1 in, 1 out]
    n145 = local read "Temperature Chart"() -> (w301:dynamicdata)
    n146 = local read "Heater Drive"() -> (w299:waveform(dbl))
    n147 = local read "Pressures"() -> (w300:waveform(dbl)[])
    n148 = Merge Signals(w301, w300, w299) -> (w303:dynamicdata)
    n149 = call "Write To Measurement File"("Signals"=w303, "Enable"="Enable", "Filename"="LogFile") -> ()  [unwired: 14 in, 3 out]
    n150 = local read "stopping"() -> (w304:bool)
    n151 = node-c288() -> ()  [unwired: 1 in, 1 out]
  }
  n152 = node-c288(w4) -> ()  [unwired: 1 out]
  n153 = call <vilib>:"Simple Error Handler.vi"("error in (no error)"=w8) -> ("error out"=w7:errorcluster)  [unwired: 4 in, 4 out]
  n154 = disable-structure shown="Default" {
    disable-tunnel: w7 -> [_ _]
    frame condition #0 (active) {
      n155 = local write "stopping"(TRUE ("stopping")) -> ()
    }
    frame condition #1 {
      # "Call Quit LabVIEW if running as a built application."
      n156 = Quit LabVIEW() -> ()  [unwired: 1 in]
    }
  }
